vi "Find Global Min on Surface.vi"() -> ()   [LabVIEW 2023]
doc: "This example demonstrates how to use the Global Optimization VI to find the global minimum on a surface. The surface is the objective function implemented by a reentrant VI that shares a clone. This example calls the Open VI Reference function to open a reference to an object function VI. It uses the 0x40 option to execute multiple cloned VIs in parallel so the Global Optimization VI can take advantage of multiple processors when evaluating the objective function.\n\nIn this example, the Global Optimization VI is in a loop and passes <b>Ending State</b> to <b>Beginning State</b> to allow a warm start of the optimization. This example returns the best minimum and all candidate minimums from <b>Ending State</b> at each loop iteration so that you can verify how the Global Optimization VI improves the candidate minimums and finds the global minimum iteratively."
uses:
  <vilib>/gmath/GlobalOptimization.llb/DE_State.ctl
  <vilib>/gmath/GlobalOptimization.llb/DE_Population.ctl
  <vilib>/gmath/GlobalOptimization.llb/DE_Settings.ctl
  <vilib>/gmath/GlobalOptimization.llb/DE_Bound Mapping Method.ctl
  <vilib>/gmath/GlobalOptimization.llb/DE_Mutation Method.ctl
  <vilib>/gmath/GlobalOptimization.llb/DE_Crossover Method.ctl
  <vilib>/gmath/GlobalOptimization.llb/DE_Stopping Criteria.ctl
  <vilib>/Utility/miscctls.llb/LVOffsetAndMultiplierTypeDef.ctl
  <vilib>/Analysis/1siggen.llb/Ramp Pattern by Samples.vi
  <vilib>/gmath/NI_AAL_GlobalOptimization.lvlib
  <vilib>/Analysis/NI_AALBase.lvlib
panel:
  out "best minimum":dbl format="%_5g"
  out "iteration":i32 min=1 max=200 step=1
  in  "number of iterations":i32=50 min=1 max=200 step=1
  in  "population size":i32=20 min=1 max=200 step=1
  out "Population":cluster{dbl[], dbl[]}(graph)
  out "Cost Function Surface":dbl[][](graph)
  # "Overview: Demonstrates the use of the Global Optimization VI to find the global minimum on a surface.\nRequirements: LabVIEW Full Development System\nInstructions:\n1. Run the VI.\n2. The Cost Function Surface graph is a visualization of the function being minimized. The best solution should end up at the lowest point of this graph.\n3. Observe how the Population members tend to cluster near the regions of lower value.  This becomes more pronounced as the iterations increase."
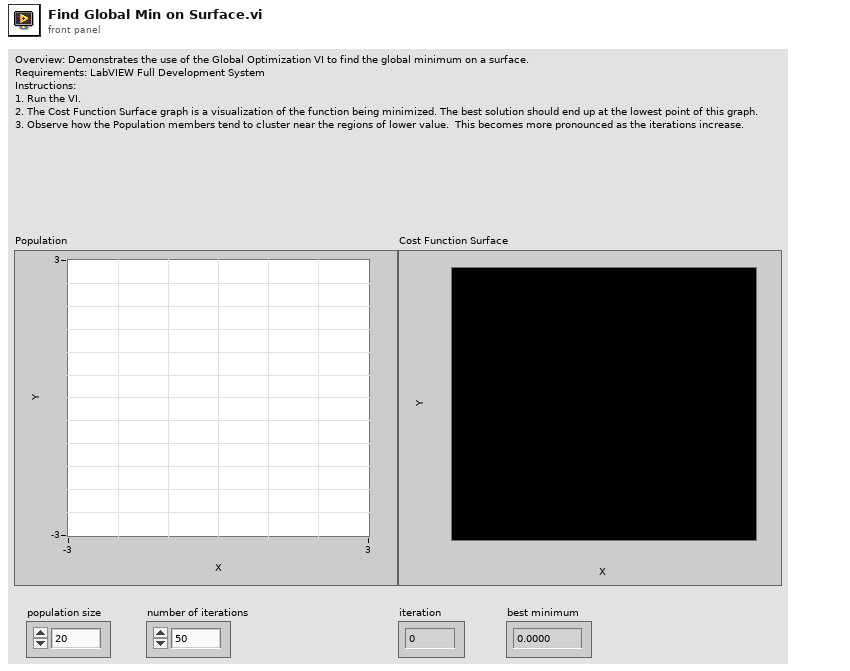
[diagram p1: front panel]
types:
  T1 = typedef "LVOffsetAndMultiplierTypeDef.ctl" = cluster{"Offset":dbl, "Multiplier":dbl}
  T2 = typedef "NI_AAL_GlobalOptimization.lvlib/DE_Stopping Criteria.ctl" = cluster{"max iterations":i32, "max function calls":i32, "max time (sec)":dbl}
  T3 = typedef "NI_AAL_GlobalOptimization.lvlib/DE_Settings.ctl" = cluster{"population size":i32, "scale factor":dbl, "crossover probability":dbl, "bound mapping method":T4, "mutation method":T5, "crossover method":T6}
  T4 = typedef "NI_AAL_GlobalOptimization.lvlib/DE_Bound Mapping Method.ctl" = u16
  T5 = typedef "NI_AAL_GlobalOptimization.lvlib/DE_Mutation Method.ctl" = u16
  T6 = typedef "NI_AAL_GlobalOptimization.lvlib/DE_Crossover Method.ctl" = u16
  T7 = typedef "NI_AAL_GlobalOptimization.lvlib/DE_State.ctl" = cluster{"Population":T8[], "Pareto Indexes":i32[]}
  T8 = typedef "NI_AAL_GlobalOptimization.lvlib/DE_Population.ctl" = cluster{"Parameters":dbl[], "Objective Functions":dbl[], "Equality Constraints":dbl[], "Inequality Constraints":dbl[]}
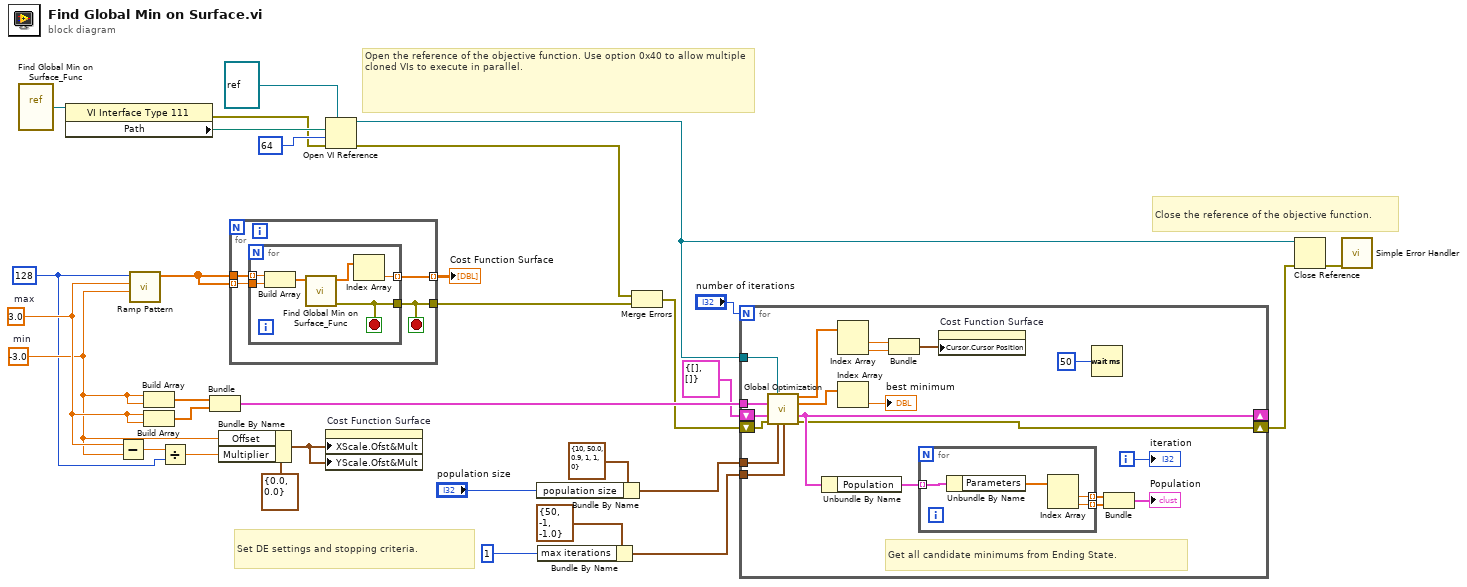
[diagram p0: block diagram]
diagram:
  w9 = 128 ("samples")
  w13 = 3.0  # max
  w11 = -3.0  # min
  # "Set DE settings and stopping criteria."
  # "Close the reference of the objective function."
  # "Open the reference of the objective function. Use option 0x40 to allow multiple cloned VIs to execute in parallel."
  n1 = vi-ref "Find Global Min on Surface_Func.vi"() -> (w6:refnum<vi>)
  n2 = property class="VI Interface Type 111"(reference=w6) -> (error out=w4:errorcluster, "Path"=w5:path)  [unwired: 1 in, 1 out]
  n3 = Subtract(x=w13, y=w11) -> (x-y=w14:dbl)
  n4 = call-poly <vilib>:"Ramp Pattern.vi"("start"=w11, "end"=w13, "samples"=w9) -> ("Ramp Pattern"=w17:dbl[])  [unwired: 7 in, 1 out]
  n5 = Build Array(w11, w11) -> (w16:dbl[])
  n6 = Build Array(w13, w13) -> (w15:dbl[])
  n7 = Divide(x=w14, y=w9) -> (x/y=w10:dbl)
  n8 = Bundle(w16, w15) -> (w31:cluster{dbl[], dbl[]})  [unwired: 1 in]
  n9 = Bundle By Name(cluster=T1 {"Offset"=0.0, "Multiplier"=0.0} ("X Scale.Offset and Multiplier"), "Offset"=w11, "Multiplier"=w10) -> (w8:T1)
  n10 = for {
    tunnel: w17 -> [w35]
    tunnel: w17 -> [w34] mode=indexing
    tunnel: [w33] -> w7 mode=indexing
    tunnel: [w32] -> w2
    stop <- w32 stop-if-true
    n11 = for {
      tunnel: w35 -> [w41] mode=indexing
      tunnel: w34 -> [w40]
      tunnel: [w37] -> w33 mode=indexing
      tunnel: [w36] -> w32
      stop <- w36 stop-if-true
      n12 = Build Array(w41, w40) -> (w39:dbl[])
      n13 = call "Find Global Min on Surface_Func.vi"("X"=w39) -> ("error out"=w36:errorcluster, "Objective Functions"=w38:dbl[])  [unwired: 7 in, 2 out]
      n14 = Index Array(array=w38) -> (element=w37:dbl)  [unwired: 1 in]
    }
  }
  "Cost Function Surface" <- w7
  n15 = Open VI Reference(type specifier VI Refnum (for type only)=refnum<vi> refnum ("objective and constraint function"), vi path=w5, options=64, error in (no error)=w4) -> (vi reference=w20:refnum<vi>, error out=w3:errorcluster)  [unwired: 2 in]
  n16 = property on="Cost Function Surface" class="IntGraph (strict)"("XScale.Ofst&Mult"=w8, "YScale.Ofst&Mult"=w8) -> ()  [unwired: 2 in, 2 out]
  n17 = Bundle By Name(cluster=T3 {"population size"=10, "scale factor"=50.0, "crossover probability"=0.9, "bound mapping method"=1, "mutation method"=1, "crossover method"=0} ("DE Settings"), "population size"="population size") -> (w28:T3)
  n18 = Bundle By Name(cluster=T2 {"max iterations"=50, "max function calls"=-1, "max time (sec)"=-1.0} ("stopping criteria"), "max iterations"=1 ("number of generations")) -> (w23:T2)
  n19 = Merge Errors(w3, w2) -> (w1:errorcluster)
  n20 = for {
    N: "number of iterations" -> [_]
    tunnel: w31 -> [w61]
    shift-right: [w55] -> _
    shift-left: T7 {"Population"=[], "Pareto Indexes"=[]} ("Ending State") -> [w56]
    tunnel: w28 -> [w49]
    tunnel: w23 -> [w48]
    tunnel: w20 -> [w46]
    shift-right: [w45] -> w19
    shift-left: w1 -> [w44]
    i -> [w47]
    # "Get all candidate minimums from Ending State."
    n21 = call <vilib>:"Global Optimization.vi"("objective and constraint function"=w46, "Bounds"=w61, "Beginning State"=w56, "error in (no error)"=w44, "DE settings"=w49, "stopping criteria"=w48) -> ("Minimum"=w60:dbl[], "F(Minimum)"=w43:dbl[], "Ending State"=w55:T7, "error out"=w45:errorcluster)  [unwired: 5 in, 1 out]
    n22 = Unbundle By Name(w55) -> ("Population"=w54:T8[])
    n23 = Index Array(array=w60) -> (element #1=w59:dbl, element #2=w58:dbl)  [unwired: 2 in]
    n24 = Index Array(array=w43) -> (element=→"best minimum":dbl)  [unwired: 1 in]
    n25 = Bundle("Numeric"=w59, "Numeric"=w58) -> (w57:cluster{"Numeric":dbl, "Numeric":dbl})  [unwired: 1 in]
    n26 = for {
      tunnel: w54 -> [w62] mode=indexing
      tunnel: [w64] -> w53 mode=indexing
      tunnel: [w63] -> w52 mode=indexing
      n27 = Unbundle By Name(w62) -> ("Parameters"=w65:dbl[])
      n28 = Index Array(array=w65) -> (element #1=w64:dbl, element #2=w63:dbl)  [unwired: 2 in]
    }
    n29 = property on="Cost Function Surface" class="IntGraph (strict)"("Cursor.Cursor Position"=w57) -> ()  [unwired: 2 in, 2 out]
    n30 = Wait (ms)(milliseconds to wait=u32 50) -> ()  [unwired: 1 out]
    n31 = Bundle(w53, w52) -> (→"Population":cluster{dbl[], dbl[]})  [unwired: 1 in]
    "iteration" <- w47
  }
  n32 = Close Reference(reference=w20, error in (no error)=w19) -> (error out=w18:errorcluster)
  n33 = call <vilib>:"Simple Error Handler.vi"("error in (no error)"=w18) -> ()  [unwired: 4 in, 5 out]
